vi "AudioStreamer.Init Output.vi"(0 "config":T2) -> (4 "Output":T1, 8 "ptsPerFrame":i32, 10 "Fs (Hz)":dbl, 12 "framesPerStim":i32, 13 "Waver mic":T1, 14 "Mic":T1, 15 "error out":errorcluster)   [LabVIEW 2020]
uses:
  Typedefs/AudioStreamer.Config.ctl
  Typedefs/AudioStreamer.Signal Specification.ctl
  <vilib>/Dataflow_G/G-Audio/Controls/Audio Device Refnum.ctl
  <vilib>/Dataflow_G/G-Audio/Controls/Audio Device Config.ctl
  <vilib>/Dataflow_G/G-Audio/Controls/Audio Device Format.ctl
  <vilib>/Dataflow_G/G-Audio/G-Audio.lvlib
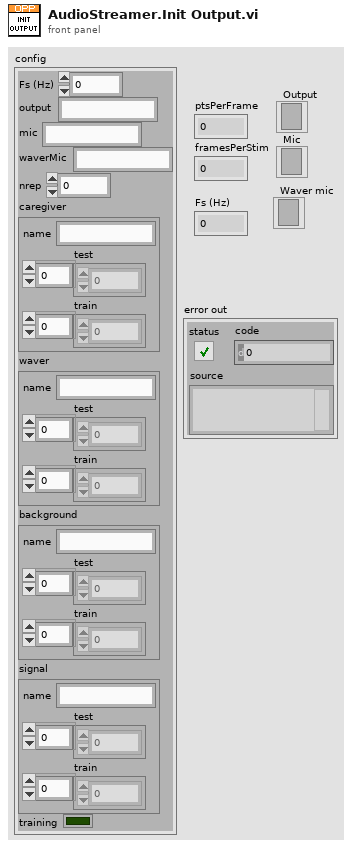
[diagram p1: front panel]
types:
  T1 = typedef "G-Audio.lvlib/Audio Device Refnum.ctl" = refnum<file>
  T2 = typedef "AudioStreamer.Config.ctl" = cluster{"Fs (Hz)":dbl, "output":string, "mic":string, "waverMic":string, "nrep":i32, "caregiver":T3, "waver":T3, "background":T3, "signal":T3, "training":bool}
  T3 = typedef "AudioStreamer.Signal Specification.ctl" = cluster{"name":string, "test":sgl[], "train":sgl[]}
  T4 = typedef "G-Audio.lvlib/Audio Device Format.ctl" = enum16{"Native", "U8", "I16", "I32", "SGL"}
  T5 = typedef "G-Audio.lvlib/Audio Device Config.ctl" = cluster{"Sample Rate (Hz)":u32, "Channels":u32, "Format":T4}
  T6 = typedef "G-Audio.lvlib/Audio Device Info.ctl" = cluster{"Name":string, "ID":u8[], "Device Type":T7, "Default":bool, "Native Data Formats":T8[]}
  T7 = typedef "G-Audio.lvlib/Audio Device Type.ctl" = enum16{"(None)", "Playback", "Capture", "Duplex", "Loopback"}
  T8 = typedef "G-Audio.lvlib/Audio Device Native Data Format.ctl" = cluster{"Format":T4, "Channels":u32, "Sample Rate (Hz)":u32, "Exclusive Mode":bool}
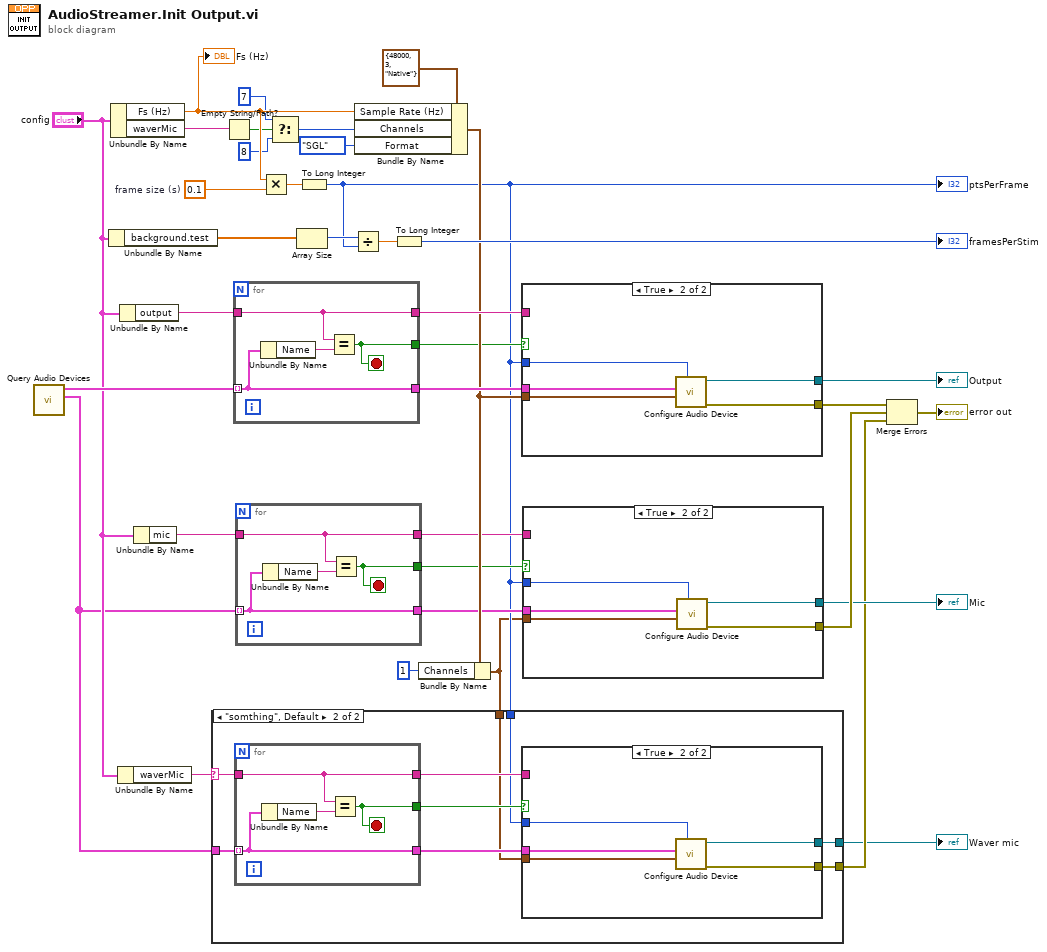
[diagram p0: block diagram]
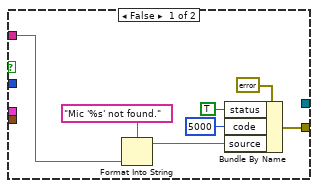
[diagram p3: hidden frame]
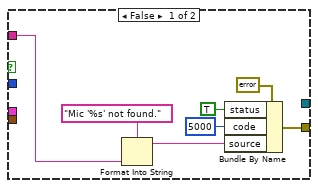
[diagram p4: hidden frame]
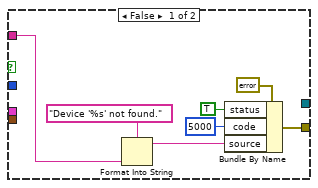
[diagram p5: hidden frame]
diagram:
  w34 = 0.1  # frame size (s)
  n1 = call <vilib>:"Query Audio Devices.vi"() -> ("Capture Devices"=w5:T6[], "Playback Devices"=w27:T6[])  [unwired: 7 in, 3 out]
  n2 = Unbundle By Name("config") -> ("background.test"=w32:sgl[])
  n3 = Unbundle By Name("config") -> ("Fs (Hz)"=w35:dbl, "waverMic"=w12:string)
  "Fs (Hz)" <- w35
  n4 = Unbundle By Name("config") -> ("waverMic"=w7:string)
  n5 = Unbundle By Name("config") -> ("output"=w28:string)
  n6 = Unbundle By Name("config") -> ("mic"=w18:string)
  n7 = Empty String/Path?(string/path=w12) -> (empty?=w11:bool)
  n8 = for {
    tunnel: w28 -> [w41]
    tunnel: [w41] -> w36
    tunnel: w27 -> [w39] mode=indexing
    tunnel: [w39] -> w26
    tunnel: [w38] -> w22
    stop <- w38 stop-if-true
    n9 = Unbundle By Name(w39) -> ("Name"=w40:string)
    n10 = Equal?(x=w41, y=w40) -> (x = y?=w38:bool)
  }
  n11 = for {
    tunnel: w18 -> [w45]
    tunnel: [w45] -> w17
    tunnel: w5 -> [w43] mode=indexing
    tunnel: [w43] -> w16
    tunnel: [w42] -> w15
    stop <- w42 stop-if-true
    n12 = Unbundle By Name(w43) -> ("Name"=w44:string)
    n13 = Equal?(x=w45, y=w44) -> (x = y?=w42:bool)
  }
  n14 = Multiply(x=w35, y=w34) -> (x*y=w33:dbl)
  n15 = Select(t=7 ("number of channels"), s=w11, f=8 ("number of channels")) -> (s? t:f=w10:i32)
  n16 = Array Size(array=w32) -> (size(s)=w31:i32)
  n17 = To Long Integer(number=w33) -> (32bit integer=w4:i32)
  "ptsPerFrame" <- w4
  n18 = Divide(x=w31, y=w4) -> (x/y=w30:dbl)
  n19 = Bundle By Name(cluster=T5 {"Sample Rate (Hz)"=48000, "Channels"=3, "Format"=enum."Native"} ("Device Config"), "Sample Rate (Hz)"=w35, "Channels"=w10, "Format"=Audio_Device_Format."SGL") -> (w23:T5)
  n20 = To Long Integer(number=w30) -> (32bit integer=→"framesPerStim":i32)
  n21 = Bundle By Name(cluster=w23, "Channels"=u32 1) -> (w3:T5)
  n22 = case shown="\"somthing\", Default" w7 {
    selector: w7 -> [_ w54]
    tunnel: w5 -> [_ w50]
    tunnel: w4 -> [_ w49]
    tunnel: w3 -> [_ w48]
    tunnel: [_ w47] -> w2
    tunnel: [_ w46] -> w1
    frame "" {
    }
    frame "somthing", Default {
      n23 = for {
        tunnel: w54 -> [w58]
        tunnel: [w58] -> w53
        tunnel: w50 -> [w56] mode=indexing
        tunnel: [w56] -> w52
        tunnel: [w55] -> w51
        stop <- w55 stop-if-true
        n24 = Unbundle By Name(w56) -> ("Name"=w57:string)
        n25 = Equal?(x=w58, y=w57) -> (x = y?=w55:bool)
      }
      n26 = case shown="True" w51 {
        tunnel: w48 -> [_ w68]
        tunnel: [w64 w69] -> w47
        tunnel: w53 -> [w61 _]
        tunnel: w52 -> [_ w70]
        tunnel: w49 -> [_ w67]
        tunnel: [_ w66] -> w46
        frame False {
          n27 = Format Into String(format string="Mic '%s' not found.", w61) -> (resulting string=w59:string)  [unwired: 2 in, 1 out]
          n28 = Bundle By Name(cluster=errorcluster {"status"=TRUE, "code"=5000, "source"=""} ("error out"), "status"=TRUE, "code"=5000, "source"=w59) -> (w64:errorcluster)
        }
        frame True {
          n29 = call <vilib>:"Configure Audio Device.vi"("Buffer Size (4096)"=w67, "Device Config"=w68, "Audio Device"=w70) -> ("error out"=w69:errorcluster, "Audio Device Refnum"=w66:T1)  [unwired: 5 in, 2 out]
        }
      }
    }
  }
  "Waver mic" <- w1
  n30 = case shown="True" w22 {
    tunnel: w23 -> [_ w80]
    tunnel: [w76 w81] -> w37
    tunnel: w36 -> [w73 _]
    tunnel: w26 -> [_ w82]
    tunnel: w4 -> [_ w79]
    tunnel: [_ w78] -> w19
    frame False {
      n31 = Format Into String(format string="Device '%s' not found.", w73) -> (resulting string=w71:string)  [unwired: 2 in, 1 out]
      n32 = Bundle By Name(cluster=errorcluster {"status"=TRUE, "code"=5000, "source"=""} ("error out"), "status"=TRUE, "code"=5000, "source"=w71) -> (w76:errorcluster)
    }
    frame True {
      n33 = call <vilib>:"Configure Audio Device.vi"("Buffer Size (4096)"=w79, "Device Config"=w80, "Audio Device"=w82) -> ("error out"=w81:errorcluster, "Audio Device Refnum"=w78:T1)  [unwired: 5 in, 2 out]
    }
  }
  "Output" <- w19
  n34 = case shown="True" w15 {
    tunnel: w3 -> [_ w92]
    tunnel: [w88 w93] -> w20
    tunnel: w17 -> [w85 _]
    tunnel: w16 -> [_ w94]
    tunnel: w4 -> [_ w91]
    tunnel: [_ w90] -> w14
    frame False {
      n35 = Format Into String(format string="Mic '%s' not found.", w85) -> (resulting string=w83:string)  [unwired: 2 in, 1 out]
      n36 = Bundle By Name(cluster=errorcluster {"status"=TRUE, "code"=5000, "source"=""} ("error out"), "status"=TRUE, "code"=5000, "source"=w83) -> (w88:errorcluster)
    }
    frame True {
      n37 = call <vilib>:"Configure Audio Device.vi"("Buffer Size (4096)"=w91, "Device Config"=w92, "Audio Device"=w94) -> ("error out"=w93:errorcluster, "Audio Device Refnum"=w90:T1)  [unwired: 5 in, 2 out]
    }
  }
  "Mic" <- w14
  n38 = Merge Errors(w37, w20, w2) -> (→"error out":errorcluster)
